vi "Write TCPClient.vi"(8 "error in (no error)":errorcluster, 10 "tcp.lvlib:TCPClient.lvclass":refnum<class "TCPClient.lvclass">, 11 "TCPClient in":refnum<class "TCPCommunication.lvclass">) -> (0 "error out":errorcluster, 3 "TCPClient out":refnum<class "TCPCommunication.lvclass">)   [LabVIEW 2016, in "TCPCommunication.lvclass"]
uses:
  TCPCommunication.lvclass
  common_ascii_tcp/TCPClient/TCPClient.lvclass
  TCPCommunication.lvclass/TCPCommunication.ctl
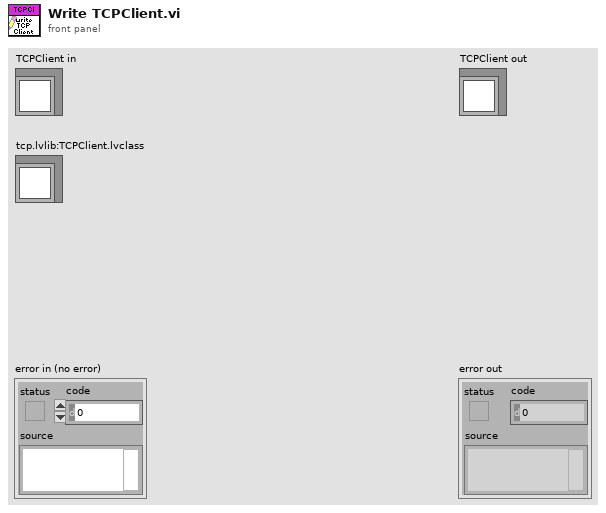
[diagram p1: front panel]
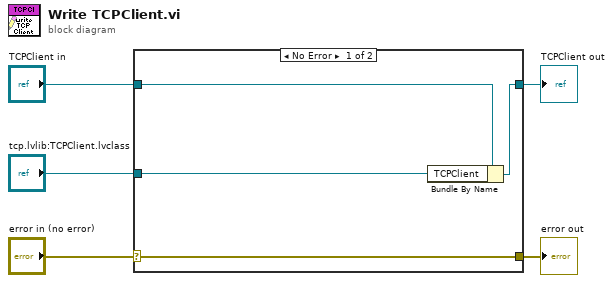
[diagram p0: block diagram]
diagram:
  n1 = case shown="No Error" "error in (no error)" {
    selector: "error in (no error)" -> [w9 w10]
    tunnel: [w9 w10] -> w4
    tunnel: [w7 w11] -> w2
    tunnel: "TCPClient in" -> [w8 w11]
    tunnel: "tcp.lvlib:TCPClient.lvclass" -> [w6 _]
    frame No Error {
      n2 = Bundle By Name(cluster=w8, "TCPClient"=w6) -> (w7:refnum<class "TCPCommunication.lvclass">)
    }
    frame Error {
    }
  }
  "error out" <- w4
  "TCPClient out" <- w2
